vi "piano UI.vi"() -> ()   [LabVIEW 2020]
uses:
  midi-file/Note Value.ctl
  midi-ui/midi-ui.lvclass
  midi/midi.lvclass
  <vilib>/Analysis/geometry.llb/Point in Polygon Position.ctl
  midi/midichannel.set.vi
  <vilib>/Analysis/geometry.llb/Point in Polygon (Scalar).vi
  midi-file/midi-file.lvclass
  <vilib>/Analysis/NI_AAL_Geometry.lvlib
panel:
  out "Data2":i32
  out "Data1":i32
  out "Status":i32
  out "Sustain":bool
  in  "Note Off":bool
  in  "Note On":bool
  in  "Note Value":T1
  out "2D Picture":picture
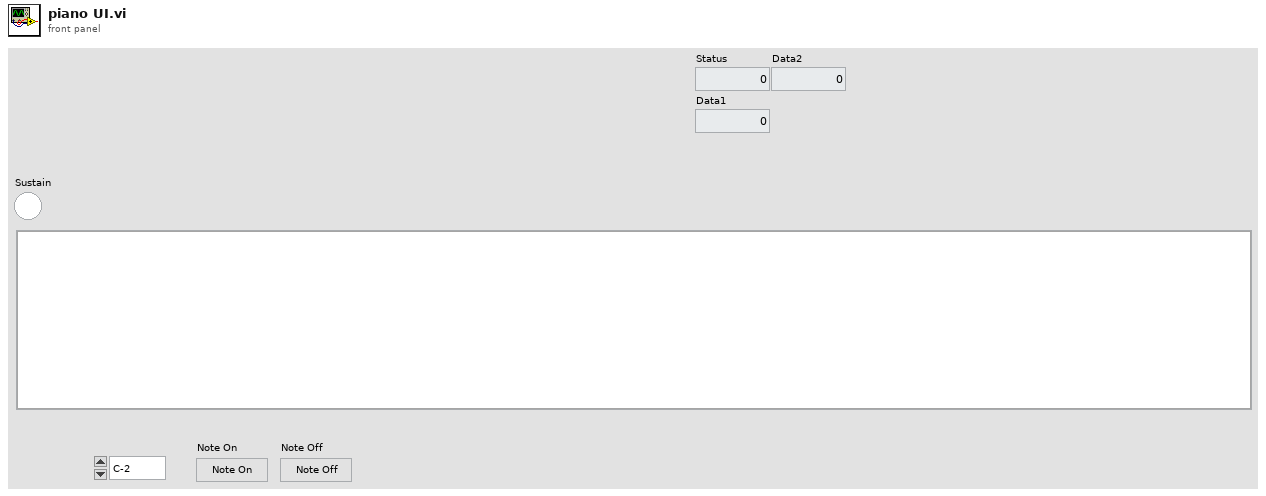
[diagram p1: front panel]
types:
  T1 = typedef "midi-file.lvclass/Note Value.ctl" = enum8{"C-2", "C#-2", "D-2", "D#-2", "E-2", "F-2", "F#-2", "G-2", "G#-2", "A-2", "A#-2", "B-2", "C-1", "C#-1", "D-1", "D#-1", "E-1", "F-1", "F#-1", "G-1", "G#-1", "A-1", "A#-1", "B-1", "C0", "C#0", "D0", "D#0", "E0", "F0", "F#0", "G0", "G#0", "A0", "A#0", "B0", "C1", "C#1", "D1", "D#1", "E1", "F1", "F#1", "G1", "G#1", "A1", "A#1", "B1", "C2", "C#2", "D2", "D#2", "E2", "F2", "F#2", "G2", "G#2", "A2", "A#2", "B2", "C3", "C#3", "D3", "D#3", "E3", "F3", "F#3", "G3", "G#3", "A3", "A#3", "B3", "C4", "C#4", "D4", "D#4", "E4", "F4", "F#4", "G4", "G#4", "A4", "A#4", "B4", "C5", "C#5", "D5", "D#5", "E5", "F5", "F#5", "G5", "G#5", "A5", "A#5", "B5", "C6", "C#6", "D6", "D#6", "E6", "F6", "F#6", "G6", "G#6", "A6", "A#6", "B6", "C7", "C#7", "D7", "D#7", "E7", "F7", "F#7", "G7", "G#7", "A7", "A#7", "B7", "C8", "C#8", "D8", "D#8", "E8", "F8", "F#8", "G"}
  T2 = cluster{"Width":u16, "Style":enum32{"Solid", "Dash", "Dot", "DashDot", "DashDotDot"}}
  T3 = typedef "LVPoint32TypeDef.ctl" = cluster{"Horizontal":i32, "Vertical":i32}
  T4 = typedef "NI_AAL_Geometry.lvlib/Point in Polygon Position.ctl" = u16
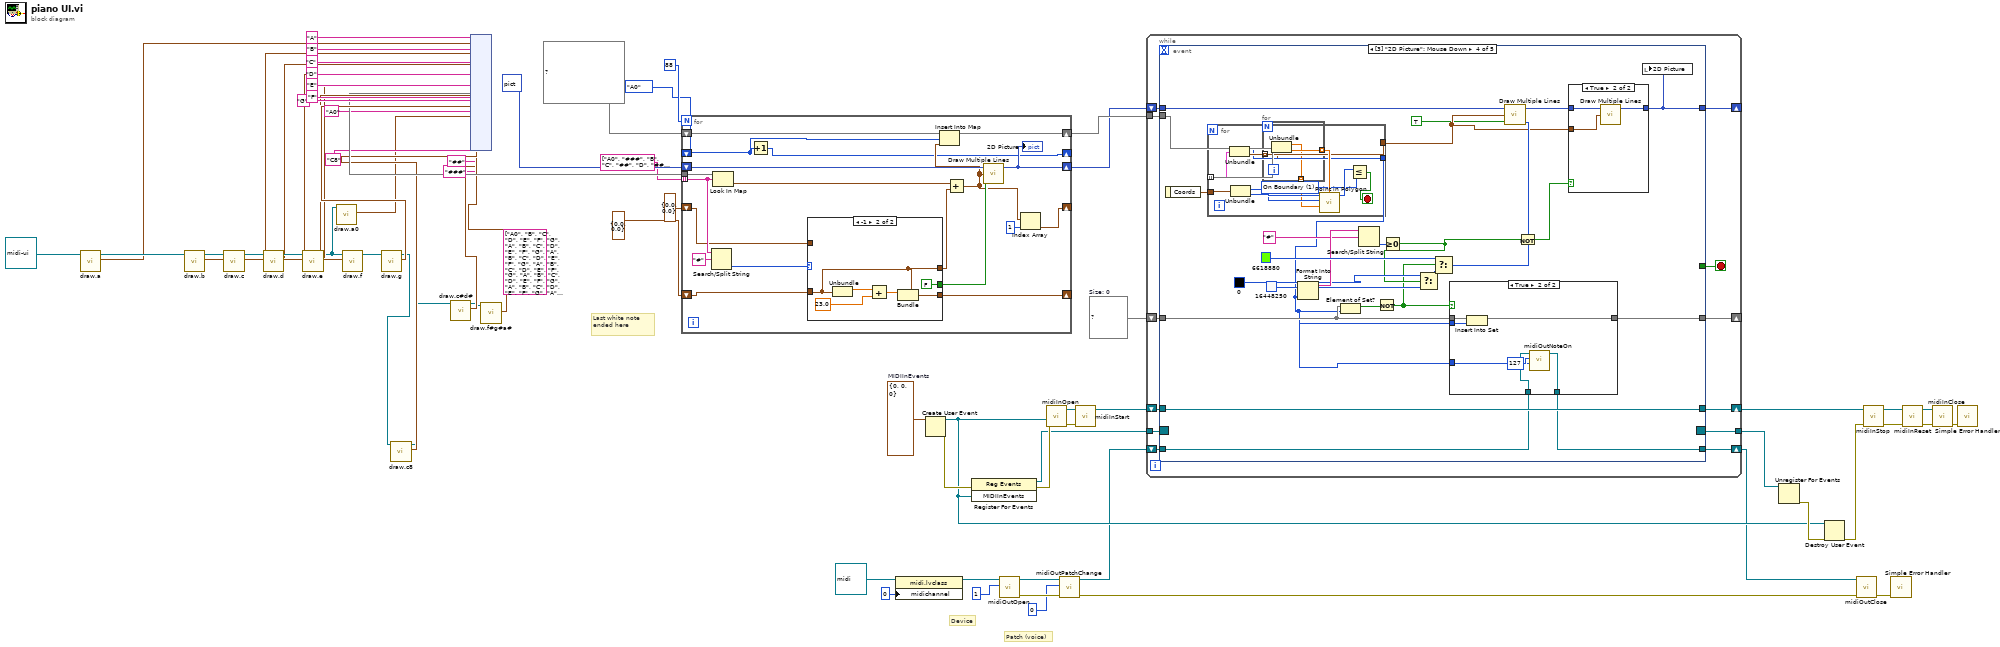
[diagram p0: block diagram]
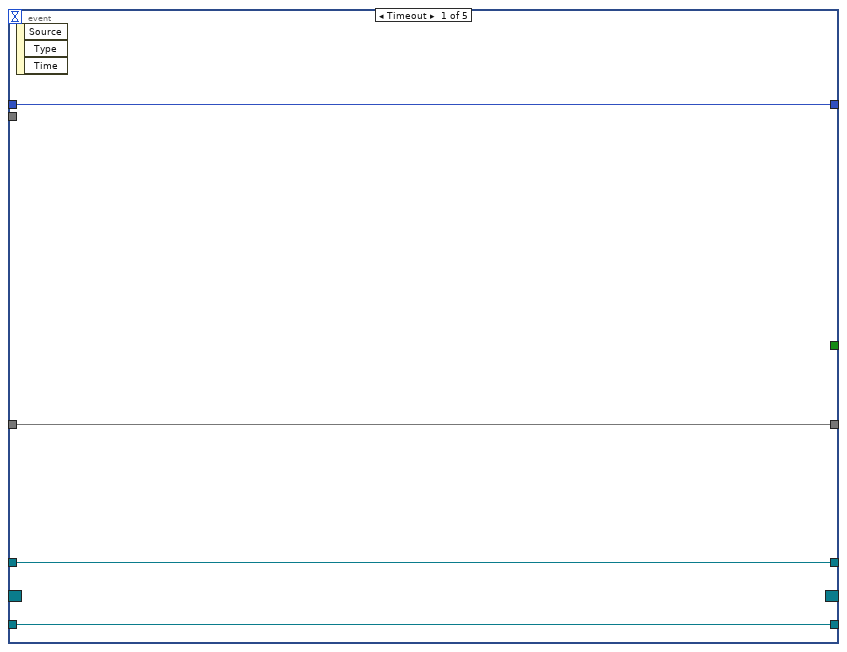
[diagram p2: hidden frame]
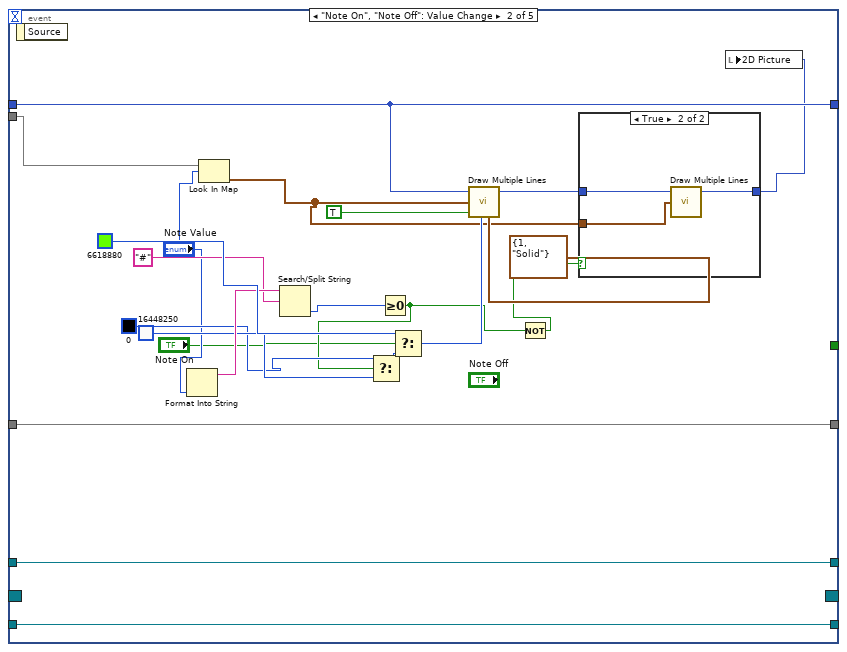
[diagram p3: hidden frame]
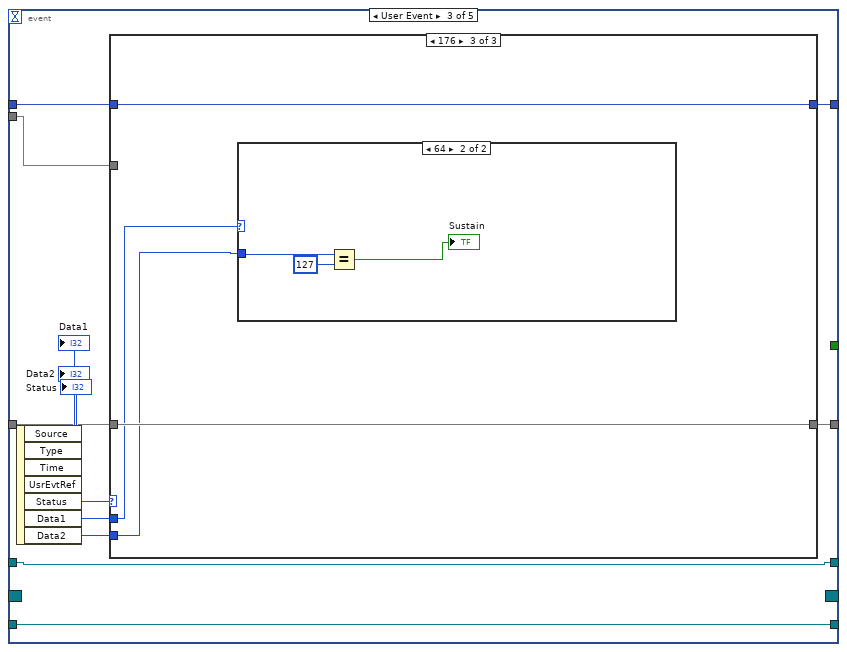
[diagram p5: hidden frame]
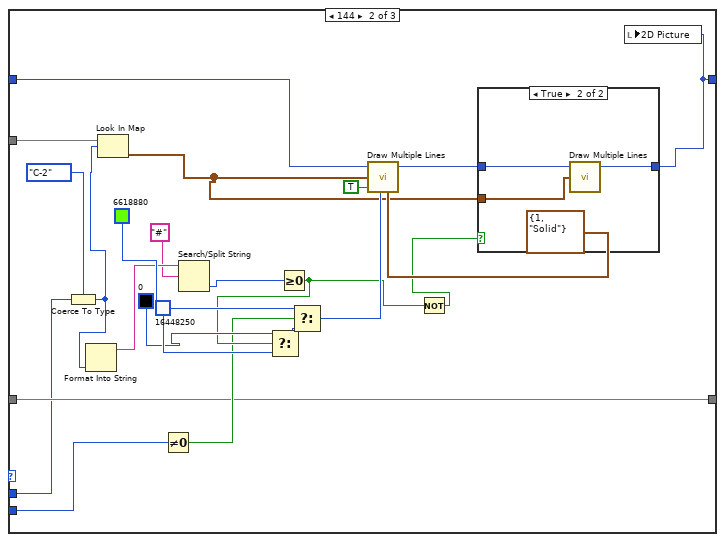
[diagram p7: hidden frame]
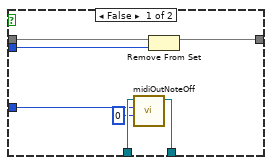
[diagram p10: hidden frame]
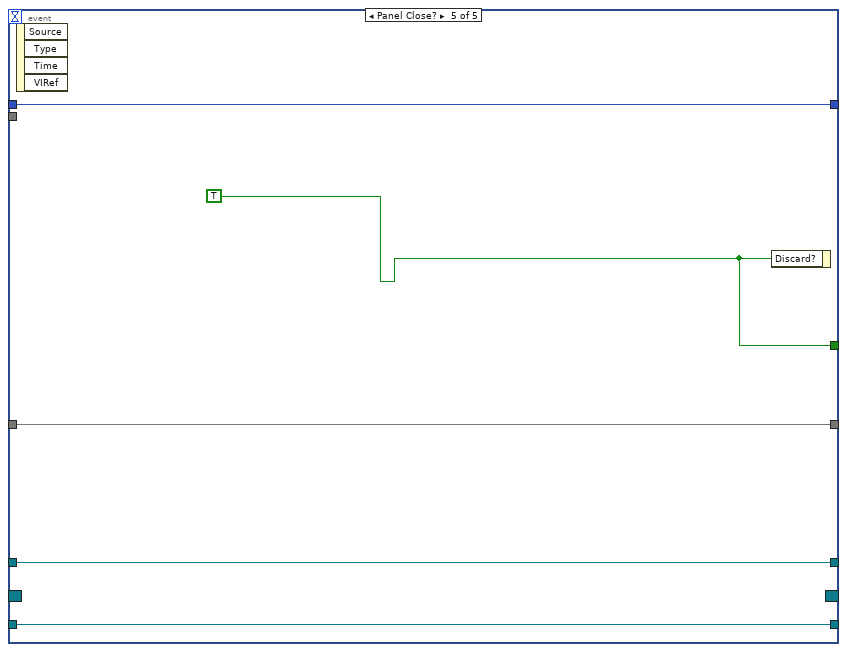
[diagram p12: hidden frame]
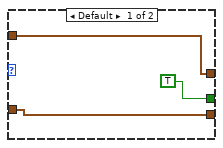
[diagram p13: hidden frame]
diagram:
  w24 = cluster{"Status":i32, "Data1":i32, "Data2":i32} {"Status"=0, "Data1"=0, "Data2"=0}  # MIDIInEvents
  w29 = set{T1} {}  # Size: 0
  (unwired) string[] ["A0", "B", "C", "D", "E", "F", "G", "A", "B", "C", "D", "E", "F", "G", "A", "B", "C", "D", "E", "F", "G", "A", "B", "C", "D", "E", "F", "G", "A", "B", "C", "D", "E", "F", "G", "A", "B", "C", "D", "E", "F", "G", "A", "B", "C", "D", "E", "F", "G", "A", "B", "C8"] ("array")
  # "Patch (voice)"
  # "Device"
  # "Last white note ended here"
  n1 = call "draw.a.vi"("midi-ui in"=refnum<class "midi-ui.lvclass"> refnum) -> ("coordinates"=w51:cluster{"x":dbl, "y":dbl}[], "midi-ui out"=w71:refnum<class "midi-ui.lvclass">)  [unwired: 9 in]
  n2 = call "draw.b.vi"("midi-ui in"=w71) -> ("coordinates"=w52:cluster{"x":dbl, "y":dbl}[], "midi-ui out"=w69:refnum<class "midi-ui.lvclass">)  [unwired: 9 in]
  n3 = call "draw.c.vi"("midi-ui in"=w69) -> ("coordinates"=w53:cluster{"x":dbl, "y":dbl}[], "midi-ui out"=w68:refnum<class "midi-ui.lvclass">)  [unwired: 9 in]
  n4 = call "draw.d.vi"("midi-ui in"=w68) -> ("coordinates"=w54:cluster{"x":dbl, "y":dbl}[], "midi-ui out"=w67:refnum<class "midi-ui.lvclass">)  [unwired: 9 in]
  n5 = call "draw.e.vi"("midi-ui in"=w67) -> ("coordinates"=w55:cluster{"x":dbl, "y":dbl}[], "midi-ui out"=w45:refnum<class "midi-ui.lvclass">)  [unwired: 9 in]
  n6 = call "draw.a0.vi"("midi-ui in"=w45) -> ("coordinates"=w44:cluster{"x":dbl, "y":dbl}[])  [unwired: 9 in, 1 out]
  n7 = call "draw.f.vi"("midi-ui in"=w45) -> ("coordinates"=w56:cluster{"x":dbl, "y":dbl}[], "midi-ui out"=w66:refnum<class "midi-ui.lvclass">)  [unwired: 9 in]
  n8 = call "draw.g.vi"("midi-ui in"=w66) -> ("coordinates"=w57:cluster{"x":dbl, "y":dbl}[], "midi-ui out"=w47:refnum<class "midi-ui.lvclass">)  [unwired: 9 in]
  n9 = call "draw.c8.vi"("midi-ui in"=w47) -> ("coordinates"=w46:cluster{"x":dbl, "y":dbl}[], "midi-ui out"=w40:refnum<class "midi-ui.lvclass">)  [unwired: 9 in]
  n10 = call "draw.c#d#.vi"("midi-ui in"=w40) -> ("coordinates"=w42:cluster{"x":dbl, "y":dbl}[], "midi-ui out"=w41:refnum<class "midi-ui.lvclass">)  [unwired: 9 in]
  n11 = call "draw.f#g#a#.vi"("midi-ui in"=w41) -> ("coordinates"=w43:cluster{"x":dbl, "y":dbl}[])  [unwired: 9 in, 1 out]
  n12 = node("A" ("key"), w51, "B" ("key"), w52, "C" ("key"), w53, "D" ("key"), w54, "E" ("key"), w55, "F" ("key"), w56, "G" ("key"), w57, "A0" ("key"), w44, "C8" ("key"), w46, "##" ("key"), w42, "###" ("key"), w43) -> (w50:map{string, cluster{"x":dbl, "y":dbl}[]})
  n13 = for {
    N: 88 -> [_]
    tunnel: w50 -> [w88]
    shift-right: [w89] -> w30
    shift-left: picture data[5B] ("picture") -> [w90]
    tunnel: string[] ["A0", "###", "B", "C", "##", "D", "##", "E", "F", "###", "G", "###", "A", "###", "B", "C", "##", "D", "##", "E", "F", "###", "G", "###", "A", "###", "B", "C", "##", "D", "##", "E", "F", "###", "G", "###", "A", "###", "B", "C", "##", "D", "##", "E", "F", "###", "G", "###", "A", "###", "B", "C", "##", "D", "##", "E", "F", "###", "G", "###", "A", "###", "B", "C", "##", "D", "##", "E", "F", "###", "G", "###", "A", "###", "B", "C", "##", "D", "##", "E", "F", "###", "G", "###", "A", "###", "B", "C8", "D", "##", "E", "F", "###", "G", "###", "A", "###", "B", "C", "##", "D", "##", "E", "F", "###", "G", "###", "A", "###", "B", "C", "##", "D", "##", "E", "F", "###", "G", "### ", ""] ("array") -> [w86] mode=indexing
    shift-right: [w83] -> _
    shift-left: cluster{"x":dbl, "y":dbl} {"x"=0.0, "y"=0.0} ("coordinate") -> [w82]
    shift-right: [w78] -> _
    shift-left: cluster{"x":dbl, "y":dbl} {"x"=0.0, "y"=0.0} ("coordinate") -> [w80]
    shift-right: [w74] -> w31
    shift-left: map{T1, cluster{"x":dbl, "y":dbl}[]} {} ("map in") -> [w75]
    shift-right: [w72] -> _
    shift-left: Note_Value."A0" ("Note Value") -> [w73]
    n14 = Search/Split String(string=w86, search string/char (-)="#") -> (offset of match=w84:i32)  [unwired: 1 in, 2 out]
    n15 = Look In Map(map=w88, key=w86) -> (value=w87:cluster{"x":dbl, "y":dbl}[])  [unwired: 1 in, 1 out]
    n16 = Increment(x=w73) -> (x+1=w72:T1)
    n17 = case shown="-1" w84 {
      tunnel: w82 -> [w93 w95]
      tunnel: [w93 w96] -> w83
      tunnel: [w92 w95] -> w81
      tunnel: w80 -> [w92 _]
      tunnel: [TRUE FALSE] -> w77
      frame Default {
      }
      frame -1 {
        n18 = Unbundle(w95) -> ("x"=w99:dbl)  [unwired: 1 out]
        n19 = Add(x=w99, y=23.0) -> (x+y=w97:dbl)
        n20 = Bundle(cluster=w95, "x"=w97) -> (w96:cluster{"x":dbl, "y":dbl})  [unwired: 1 in]
      }
    }
    n21 = Add(x=w87, y=w81) -> (x+y=w76:cluster{"x":dbl, "y":dbl}[])
    n22 = Insert Into Map(map in=w75, key=w73, value=w76) -> (map out=w74:map{T1, cluster{"x":dbl, "y":dbl}[]})  [unwired: 2 out]
    n23 = call <vilib>:"Draw Multiple Lines.vi"("picture"=w90, "line endpoints"=w76, "fill?(F)"=w77) -> ("new picture"=w89:picture)  [unwired: 6 in]
    "2D Picture" <- w89
    n24 = Index Array(array=w76, index=1) -> (element=w78:cluster{"x":dbl, "y":dbl})
  }
  n25 = property class="midi.lvclass"(reference=refnum<class "midi.lvclass"> refnum ("midi in"), "midichannel"=u64 0) -> (reference out=w4:refnum<class "midi.lvclass">)  [unwired: 1 in, 1 out]
  n26 = Create User Event(user event datatype=w24) -> (user event=w12:refnum<user-event>, error out=w26:errorcluster)  [unwired: 1 in]
  n27 = register-events(error in=w26, w12) -> (reference out=w14:refnum<event-registration>, error out=w27:errorcluster)  [unwired: 1 in]
  n28 = call "midiOutOpen.vi"("DeviceID"=u32 1, "midi in"=w4) -> ("error out"=w8:errorcluster, "midi out"=w9:refnum<class "midi.lvclass">)  [unwired: 8 in]
  n29 = call "midiInOpen.vi"("error in"=w27, "MidiDataEvents"=w12) -> ("error out"=w17:errorcluster, "midi out"=w18:refnum<class "midi.lvclass">)  [unwired: 8 in]
  n30 = call "midiOutPatchChange.vi"("error in"=w8, "Patch"=u32 0, "midi in"=w9) -> ("error out"=w1:errorcluster, "midi out"=w3:refnum<class "midi.lvclass">)  [unwired: 7 in]
  n31 = call "midiInStart.vi"("error in"=w17, "midi in"=w18) -> ("midi out"=w16:refnum<class "midi.lvclass">)  [unwired: 8 in, 1 out]
  n32 = while {
    tunnel: w31 -> [w111]
    shift-right: [w107] -> _
    shift-left: w29 -> [w108]
    shift-right: [w106] -> _
    shift-left: w30 -> [w110]
    shift-right: [w104] -> w15
    shift-left: w16 -> [w105]
    tunnel: w14 -> [w103]
    tunnel: [w102] -> w13
    shift-right: [w100] -> w2
    shift-left: w3 -> [w101]
    stop <- w109 stop-if-true
    n33 = event shown="[3] \"2D Picture\": Mouse Down" {
      selector: w103 -> [_ _ _ _ _]
      dyn-events: [_ _ _ _ _] -> w102
      timeout: _ -> [_ _ _ _ _]
      tunnel: w111 -> [_ w137 w151 w201 _]
      tunnel: w110 -> [w114 w136 w150 w212 w247]
      tunnel: [_ _ _ _ w249] -> w109
      tunnel: w108 -> [w115 w120 w144 w196 w248]
      tunnel: [w115 w120 w145 w195 w248] -> w107
      tunnel: [w114 w136 w143 w194 w247] -> w106
      tunnel: w105 -> [w113 w117 w146 w191 w246]
      tunnel: [w113 w117 w146 w191 w246] -> w104
      tunnel: w101 -> [w112 w116 w142 w190 w245]
      tunnel: [w112 w116 w142 w189 w245] -> w100
      event Timeout {
        n34 = event-data() -> ()  [unwired: 1 in, 3 out]
      }
      event "Note On", "Note Off": Value Change {
        n35 = event-data() -> ()  [unwired: 1 in, 1 out]
        n36 = Format Into String("Note Value") -> (resulting string=w133:string)  [unwired: 3 in, 1 out]
        n37 = Look In Map(map=w137, key="Note Value") -> (value=w123:cluster{"x":dbl, "y":dbl}[])  [unwired: 1 in, 1 out]
        n38 = Search/Split String(string=w133, search string/char (-)="#") -> (offset of match=w131:i32)  [unwired: 1 in, 2 out]
        n39 = Greater Or Equal To 0?(x=w131) -> (x >= 0?=w122:bool)
        n40 = Select(t=u32 0 ("color(black)"), s=w122, f=u32 16448250 ("color(black)")) -> (s? t:f=w128:u32)
        n41 = Select(t=u32 6618880 ("color(black)"), s="Note On", f=w128) -> (s? t:f=w134:u32)
        n42 = call <vilib>:"Draw Multiple Lines.vi"("picture"=w136, "line endpoints"=w123, "fill?(F)"=TRUE, "color(black)"=w134, "pen"=T2 {"Width"=1, "Style"=enum."Solid"}) -> ("new picture"=w124:picture)  [unwired: 4 in]
        n43 = Not(x=w122) -> (.not. x?=w121:bool)
        n44 = case shown="True" w121 {
          tunnel: [w138 w140] -> w125
          tunnel: w124 -> [w138 w141]
          tunnel: w123 -> [_ w139]
          frame False {
          }
          frame True {
            n45 = call <vilib>:"Draw Multiple Lines.vi"("picture"=w141, "line endpoints"=w139) -> ("new picture"=w140:picture)  [unwired: 7 in]
          }
        }
        n46 = local write "2D Picture"(w125) -> ()
      }
      event User Event {
        n47 = event-data() -> ("Status"=w147:i32, "Data1"=w149:i32, "Data2"=w148:i32)  [unwired: 1 in, 4 out]
        "Status" <- w147
        "Data1" <- w149
        "Data2" <- w148
        n48 = case shown="176" w147 {
          tunnel: w151 -> [_ w176 _]
          tunnel: w150 -> [w152 w175 w183]
          tunnel: w149 -> [_ w155 w182]
          tunnel: w148 -> [_ w159 w181]
          tunnel: [w153 w158 w184] -> w145
          tunnel: w144 -> [w153 w158 w184]
          tunnel: [w152 w157 w183] -> w143
          frame 0, Default {
          }
          frame 144 {
            n49 = Coerce To Type(0:w155, 1:Note_Value."C-2" ("key")) -> (2:w154:T1)
            n50 = Format Into String(w154) -> (resulting string=w172:string)  [unwired: 3 in, 1 out]
            n51 = Look In Map(map=w176, key=w154) -> (value=w164:cluster{"x":dbl, "y":dbl}[])  [unwired: 1 in, 1 out]
            n52 = Not Equal To 0?(x=w159) -> (x != 0?=w160:bool)
            n53 = Search/Split String(string=w172, search string/char (-)="#") -> (offset of match=w170:i32)  [unwired: 1 in, 2 out]
            n54 = Greater Or Equal To 0?(x=w170) -> (x >= 0?=w163:bool)
            n55 = Select(t=u32 0 ("color(black)"), s=w163, f=u32 16448250 ("color(black)")) -> (s? t:f=w167:u32)
            n56 = Select(t=u32 6618880 ("color(black)"), s=w160, f=w167) -> (s? t:f=w173:u32)
            n57 = call <vilib>:"Draw Multiple Lines.vi"("picture"=w175, "line endpoints"=w164, "fill?(F)"=TRUE, "color(black)"=w173, "pen"=T2 {"Width"=1, "Style"=enum."Solid"}) -> ("new picture"=w165:picture)  [unwired: 4 in]
            n58 = Not(x=w163) -> (.not. x?=w162:bool)
            n59 = case shown="True" w162 {
              tunnel: [w177 w179] -> w157
              tunnel: w165 -> [w177 w180]
              tunnel: w164 -> [_ w178]
              frame False {
              }
              frame True {
                n60 = call <vilib>:"Draw Multiple Lines.vi"("picture"=w180, "line endpoints"=w178) -> ("new picture"=w179:picture)  [unwired: 7 in]
              }
            }
            n61 = local write "2D Picture"(w157) -> ()
          }
          frame 176 {
            n62 = case shown="64" w182 {
              tunnel: w181 -> [_ w187]
              frame 0, Default {
              }
              frame 64 {
                n63 = Equal?(x=w187, y=127) -> (x = y?=→"Sustain":bool)
              }
            }
          }
        }
      }
      event "2D Picture": Mouse Down {
        n64 = event-data() -> ("Coords"=w200:T3)  [unwired: 1 in]
        n65 = for {
          tunnel: w201 -> [w234] mode=indexing
          tunnel: w200 -> [w237]
          tunnel: [w228] -> w199
          tunnel: [w227] -> w188
          stop <- w229 stop-if-true
          w230 = T4 1 items=["Inside", "On Boundary", "Outside"] ("y")
          n66 = Unbundle(w234) -> ("Note Value"=w227:T1, w228:cluster{"x":dbl, "y":dbl}[])
          n67 = Unbundle(w237) -> ("Horizontal"=w236:i32, "Vertical"=w235:i32)
          n68 = for {
            tunnel: w228 -> [w240] mode=indexing
            tunnel: [w239] -> w232 mode=indexing
            tunnel: [w238] -> w233 mode=indexing
            n69 = Unbundle(w240) -> ("x"=w238:dbl, "y"=w239:dbl)
          }
          n70 = call-poly <vilib>:"Point in Polygon.vi"("Polygon Y"=w232, "Polygon X"=w233, "y"=w235, "x"=w236) -> ("position"=w231:T4)  [unwired: 6 in, 1 out]
          n71 = Less Or Equal?(x=w231, y=w230) -> (x <= y?=w229:bool)
        }
        n72 = Format Into String(w188) -> (resulting string=w209:string)  [unwired: 3 in, 1 out]
        n73 = Element of Set?(10:w188, 11:w196) -> (3:w197:bool)
        n74 = Search/Split String(string=w209, search string/char (-)="#") -> (offset of match=w207:i32)  [unwired: 1 in, 2 out]
        n75 = Not(x=w197) -> (.not. x?=w193:bool)
        n76 = Greater Or Equal To 0?(x=w207) -> (x >= 0?=w198:bool)
        n77 = Select(t=u32 0 ("color(black)"), s=w198, f=u32 16448250 ("color(black)")) -> (s? t:f=w204:u32)
        n78 = Select(t=u32 6618880 ("color(black)"), s=w193, f=w204) -> (s? t:f=w210:u32)
        n79 = case shown="True" w193 {
          tunnel: w196 -> [w219 w226]
          tunnel: [w217 w225] -> w195
          tunnel: w188 -> [w218 w224]
          tunnel: w190 -> [w216 w223]
          tunnel: [w215 w222] -> w189
          tunnel: w188 -> [w214 w221]
          frame False {
            n80 = call "midiOutNoteOff.vi"("Velocity (0-127)"=0, "Note (0-127)"=w214, "midi in"=w216) -> ("midi out"=w215:refnum<class "midi.lvclass">)  [unwired: 7 in, 1 out]
            n81 = Remove From Set(10:w218, 11:w219) -> (3:w217:set{T1})  [unwired: 1 out]
          }
          frame True {
            n82 = Insert Into Set(10:w224, 11:w226) -> (3:w225:set{T1})  [unwired: 1 out]
            n83 = call "midiOutNoteOn.vi"("Velocity (0-127)"=127, "Note (0-127)"=w221, "midi in"=w223) -> ("midi out"=w222:refnum<class "midi.lvclass">)  [unwired: 7 in, 1 out]
          }
        }
        n84 = call <vilib>:"Draw Multiple Lines.vi"("picture"=w212, "line endpoints"=w199, "fill?(F)"=TRUE, "color(black)"=w210) -> ("new picture"=w203:picture)  [unwired: 5 in]
        n85 = Not(x=w198) -> (.not. x?=w202:bool)
        n86 = case shown="True" w202 {
          tunnel: [w241 w243] -> w194
          tunnel: w203 -> [w241 w244]
          tunnel: w199 -> [_ w242]
          frame False {
          }
          frame True {
            n87 = call <vilib>:"Draw Multiple Lines.vi"("picture"=w244, "line endpoints"=w242) -> ("new picture"=w243:picture)  [unwired: 7 in]
          }
        }
        n88 = local write "2D Picture"(w194) -> ()
      }
      event Panel Close? {
        w249 = TRUE
        n89 = event-data() -> ()  [unwired: 1 in, 4 out]
        n90 = event-data("Discard?"=w249) -> ()  [unwired: 1 in, 1 out]
      }
    }
  }
  n91 = Unregister For Events(event registration refnum=w13) -> (error out=w28:errorcluster)  [unwired: 1 in]
  n92 = Destroy User Event(user event=w12, error in=w28) -> (error out=w23:errorcluster)
  n93 = call "midiOutClose.vi"("error in"=w1, "midi in"=w2) -> ("error out"=w11:errorcluster)  [unwired: 8 in, 1 out]
  n94 = call "midiInStop.vi"("error in"=w23, "midi in"=w15) -> ("error out"=w22:errorcluster, "midi out"=w21:refnum<class "midi.lvclass">)  [unwired: 8 in]
  n95 = call <vilib>:"Simple Error Handler.vi"("error in (no error)"=w11) -> ()  [unwired: 4 in, 5 out]
  n96 = call "midiInReset.vi"("error in"=w22, "midi in"=w21) -> ("error out"=w20:errorcluster, "midi out"=w19:refnum<class "midi.lvclass">)  [unwired: 8 in]
  n97 = call "midiInClose.vi"("error in"=w20, "midi in"=w19) -> ("error out"=w25:errorcluster)  [unwired: 8 in, 1 out]
  n98 = call <vilib>:"Simple Error Handler.vi"("error in (no error)"=w25) -> ()  [unwired: 4 in, 5 out]
